vi "Format String for CSV.vi"(11 "Row Data":string[](array[string])) -> (3 "CSV Formatted strings":string[](array[string]))   [LabVIEW 2022 SP3, in "CSV Export.lvlib" / "CSV Export.lvclass"]
uses:
  CSV Export.lvclass
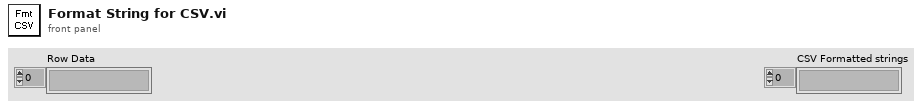
[diagram p1: front panel]
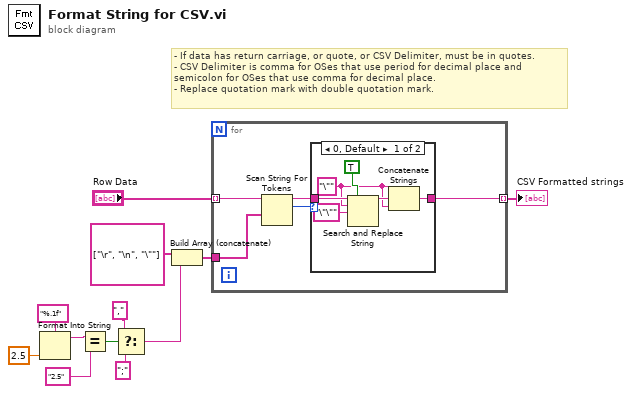
[diagram p0: block diagram]
diagram:
  # "- If data has return carriage, or quote, or CSV Delimiter, must be in quotes.\n- CSV Delimiter is comma for OSes that use period for decimal place and semicolon for OSes that use comma for decimal place.\n- Replace quotation mark with double quotation mark."
  n1 = Format Into String(format string="%.1f", 2.5 ("input 1")) -> (resulting string=w10:string)  [unwired: 2 in, 1 out]
  n2 = Equal?(x=w10, y="2.5") -> (x = y?=w7:bool)
  n3 = Select(t=",", s=w7, f=";") -> (s? t:f=w3:string)
  n4 = Build Array (concatenate)(string[] ["\r", "\n", "\""] ("operators (none)"), w3) -> (w4:string[])
  n5 = for {
    tunnel: "Row Data" -> [w14] mode=indexing
    tunnel: w4 -> [w16]
    tunnel: [w13] -> w1 mode=indexing
    n6 = Scan String For Tokens(7:w16, 9:w14) -> (2:w15:i32)  [unwired: 4 in, 3 out]
    n7 = case shown="0, Default" w15 {
      tunnel: w14 -> [w22 w23]
      tunnel: [w18 w23] -> w13
      frame 0, Default {
        w17 = "\"" ("search string")
        n8 = Search and Replace String(replace all?=TRUE ("replace all? (F)"), input string=w22, search string=w17, replace string="\"\"" ("replace string (\"\")")) -> (result string=w19:string)  [unwired: 4 in, 3 out]
        n9 = Concatenate Strings(w17, w19, w17) -> (w18:string)
      }
      frame -1 {
        # "No special chars"
      }
    }
  }
  "CSV Formatted strings" <- w1
